vi "JH z-slider motor down-up loop.vi"() -> ()   [LabVIEW 2014]
uses:
  <userlib>/Nanonis Prog Interface V5/Nanonis Prog Interface.lvlib
panel:
  out "down count 2":i32
  in  "down arrow presses 2":u16=1
  in  "down Ampltidue (V) 2":sgl=nan
  in  "down Frequency (Hz) 2":sgl=1000.0
  in  "down steps 2":u16=2000
  out "up count 2":i32
  in  "up steps 2":u16=2000
  in  "up arrow presses 2":u16=1
  in  "up Amplitude (V) 2":sgl=nan
  in  "up Frequency (Hz) 2":sgl=1000.0
  out "up count":i32
  out "down count":i32
  in  "up steps":u16=2000
  in  "up arrow presses":u16=1
  in  "up Amplitude (V)":sgl=nan
  in  "up Frequency (Hz)":sgl=1000.0
  in  "down arrow presses":u16=1
  in  "down Ampltidue (V)":sgl=nan
  in  "down Frequency (Hz)":sgl=1000.0
  in  "down steps":u16=2000
  in  "stop":bool
  out "lap count":i32
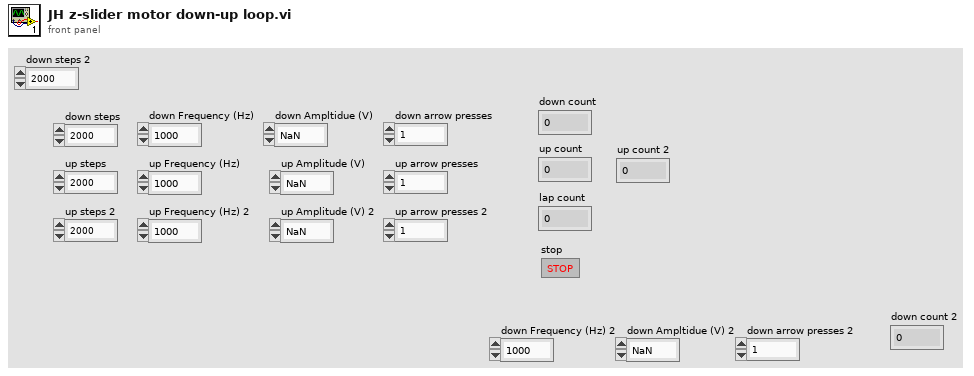
[diagram p1: front panel]
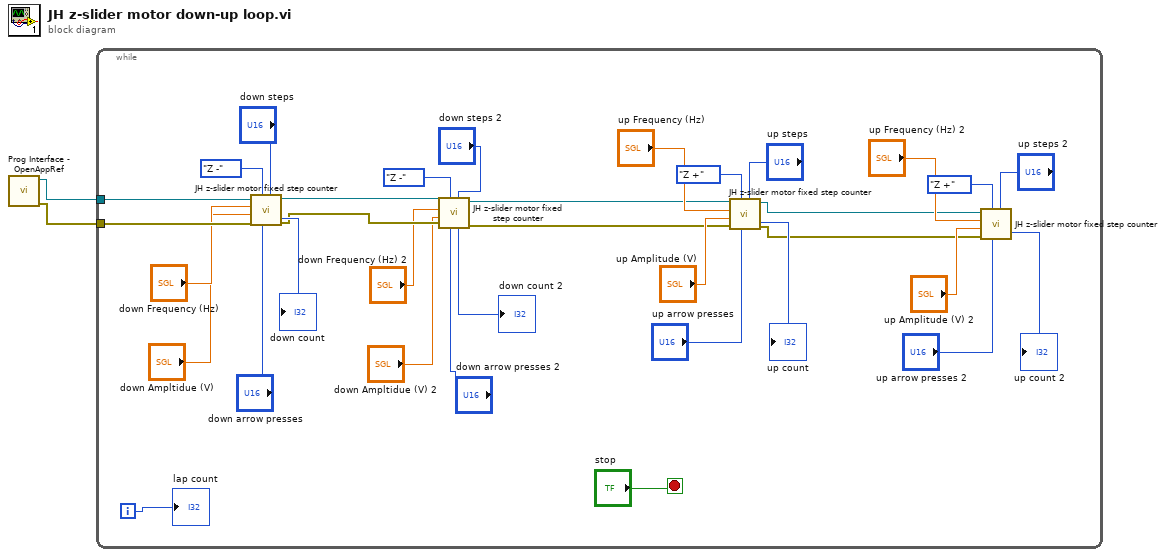
[diagram p0: block diagram]
diagram:
  n1 = call <userlib>:"Prog Interface - OpenAppRef.vi"() -> ("Error out"=w1:errorcluster, "Application reference"=w2:refnum<vi>)  [unwired: 6 in]
  n2 = while {
    tunnel: w2 -> [w34]
    tunnel: w1 -> [w33]
    i -> [w36]
    stop <- "stop" stop-if-true
    n3 = call "JH z-slider motor fixed step counter.vi"("Number of steps"="down steps", "arrow presses"="down arrow presses", "Direction"=enum16{"X +", "X -", "Y +", "Y -", "Z +", "Z -"}."Z -", "Error in (no error)"=w33, "Amplitude (V) (NaN=no change)"="down Ampltidue (V)", "Frequency (Hz) (NaN=no change)"="down Frequency (Hz)", "Application ref in"=w34) -> ("Error out"=w10:errorcluster, "Application ref out"=w12:refnum<vi>, "press counter"=→"down count":i32)  [unwired: 2 in]
    n4 = call "JH z-slider motor fixed step counter.vi"("Number of steps"="down steps 2", "arrow presses"="down arrow presses 2", "Direction"=enum16{"X +", "X -", "Y +", "Y -", "Z +", "Z -"}."Z -", "Error in (no error)"=w10, "Amplitude (V) (NaN=no change)"="down Ampltidue (V) 2", "Frequency (Hz) (NaN=no change)"="down Frequency (Hz) 2", "Application ref in"=w12) -> ("Error out"=w5:errorcluster, "Application ref out"=w11:refnum<vi>, "press counter"=→"down count 2":i32)  [unwired: 2 in]
    n5 = call "JH z-slider motor fixed step counter.vi"("Number of steps"="up steps", "arrow presses"="up arrow presses", "Direction"=enum16{"X +", "X -", "Y +", "Y -", "Z +", "Z -"}."Z +", "Error in (no error)"=w5, "Amplitude (V) (NaN=no change)"="up Amplitude (V)", "Frequency (Hz) (NaN=no change)"="up Frequency (Hz)", "Application ref in"=w11) -> ("Error out"=w13:errorcluster, "Application ref out"=w14:refnum<vi>, "press counter"=→"up count":i32)  [unwired: 2 in]
    n6 = call "JH z-slider motor fixed step counter.vi"("Number of steps"="up steps 2", "arrow presses"="up arrow presses 2", "Direction"=enum16{"X +", "X -", "Y +", "Y -", "Z +", "Z -"}."Z +", "Error in (no error)"=w13, "Amplitude (V) (NaN=no change)"="up Amplitude (V) 2", "Frequency (Hz) (NaN=no change)"="up Frequency (Hz) 2", "Application ref in"=w14) -> ("press counter"=→"up count 2":i32)  [unwired: 2 in, 2 out]
    "lap count" <- w36
  }
